vi "Create connection object.vi"(8 "error in (no error)":errorcluster, 10 "db handle":u64, 11 "SQLite dll":path) -> (0 "error out":errorcluster, 3 "Connection out":refnum<class "Connection.lvclass">)   [LabVIEW 2011, in "SQLite.lvlib" / "Connection.lvclass"]
uses:
  Connection.lvclass
  Connection.lvclass/Connection.ctl
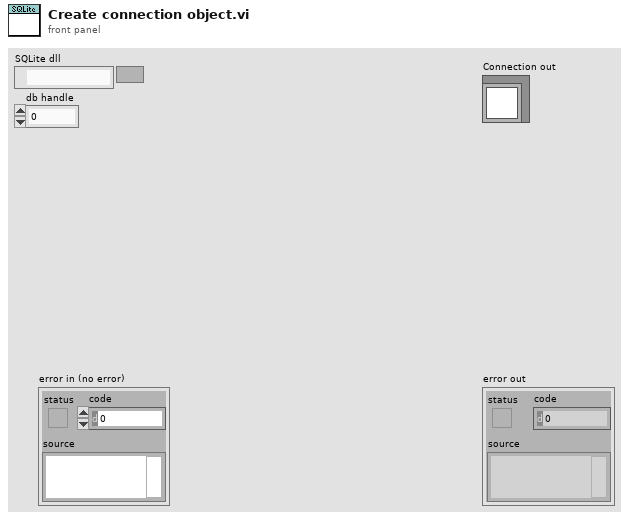
[diagram p1: front panel]
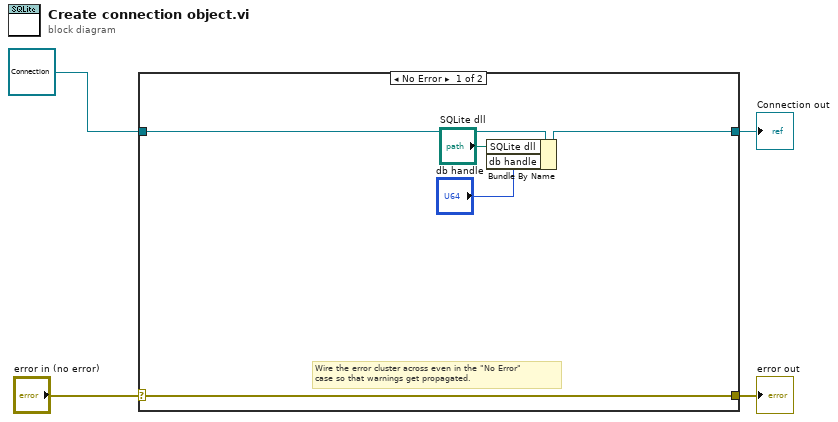
[diagram p0: block diagram]
diagram:
  n1 = case shown="No Error" "error in (no error)" {
    selector: "error in (no error)" -> [w8 w11]
    tunnel: [w8 w11] -> w3
    tunnel: [w7 w10] -> w1
    tunnel: refnum<class "Connection.lvclass"> refnum ("Connection in") -> [w9 w10]
    frame No Error {
      # "Wire the error cluster across even in the \"No Error\"\ncase so that warnings get propagated."
      n2 = Bundle By Name(cluster=w9, "SQLite dll"="SQLite dll", "db handle"="db handle") -> (w7:refnum<class "Connection.lvclass">)
    }
    frame Error {
    }
  }
  "error out" <- w3
  "Connection out" <- w1
